vi "Set Control with Signaling.vi"(5 "vi reference":refnum<vi>, 6 "Machine Name":string, 7 "Target LV Version #":T1, 8 "error in (no error)":errorcluster, 9 "Value":variant, 10 "Control Name":string="Client", 11 "VI Name":string="Client with Signaling") -> (0 "error out":errorcluster)   [LabVIEW 2020]
uses:
  Sub Controls/LV Versions Enum.ctl
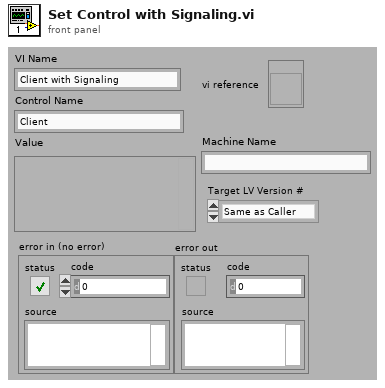
[diagram p1: front panel]
types:
  T1 = typedef "LV Versions Enum.ctl" = enum16{"Same as Caller", "8.0", "8.20", "8.5", "8.6", "9.0", "10.0", "11.0", "12.0", "13.0", "14.0", "15.0", "16.0", "17.0", "18.0", "19.0", "20.0"}
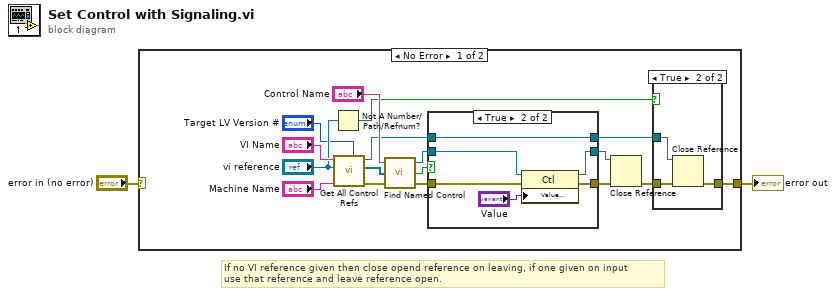
[diagram p0: block diagram]
diagram:
  # "If no VI reference given then close opend reference on leaving, if one given on input\nuse that reference and leave reference open."
  n1 = case shown="No Error" "error in (no error)" {
    selector: "error in (no error)" -> [_ w33]
    tunnel: [w6 w33] -> w2
    frame No Error {
      n2 = Not A Number/Path/Refnum?(number/path/refnum="vi reference") -> (NaN/Path/Refnum?=w4:bool)
      n3 = call "Get All Control Refs.vi"("VI Name"="VI Name", "vi reference"="vi reference", "Machine Name"="Machine Name", "Target LV Version #"="Target LV Version #") -> ("VI Refnum"=w8:refnum<vi>, "All Controls"=w15:refnum<vi>[], "error out"=w14:errorcluster)  [unwired: 2 in]
      n4 = call "Find Named Control.vi"("error in"=w14, "All Controls"=w15, "Control Name"="Control Name") -> ("error out"=w10:errorcluster, "Found"=w11:bool, "Ctl Refnum"=w12:refnum<vi>)
      n5 = case shown="True" w11 {
        tunnel: w12 -> [w25 w31]
        tunnel: [w25 w30] -> w19
        tunnel: [w26 w29] -> w18
        tunnel: w10 -> [w26 w28]
        tunnel: w8 -> [w24 w27]
        tunnel: [w24 w27] -> w9
        frame False {
        }
        frame True {
          n6 = property class="Ctl"(reference=w31, error in=w28, "Value (Signaling)"="Value") -> (reference out=w30:refnum<vi>, error out=w29:errorcluster)
        }
      }
      n7 = Close Reference(reference=w19, error in (no error)=w18) -> (error out=w7:errorcluster)
      n8 = case shown="True" w4 {
        tunnel: w9 -> [_ w23]
        tunnel: w7 -> [w20 w22]
        tunnel: [w20 w21] -> w6
        frame False {
        }
        frame True {
          n9 = Close Reference(reference=w23, error in (no error)=w22) -> (error out=w21:errorcluster)
        }
      }
    }
    frame Error {
    }
  }
  "error out" <- w2
